vi "New.vi"(8 "Error In":errorcluster) -> (0 "Error Out":errorcluster, 3 "String":refnum<class "String.lvclass">)   [LabVIEW 2018]
uses:
  String.lvclass
  D:/Users/cfield/Code/Field R&D Services/Mustache/trunk/src/Toolkit/Writers/Abstract/Abstract.lvclass
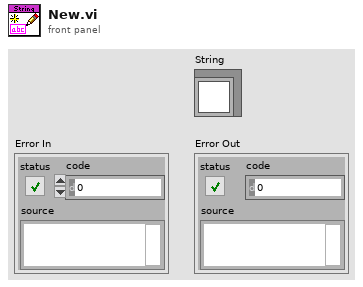
[diagram p1: front panel]
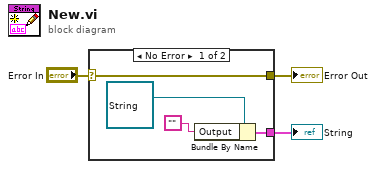
[diagram p0: block diagram]
diagram:
  n1 = case shown="No Error" "Error In" {
    selector: "Error In" -> [w4 w8]
    tunnel: [w6 _] -> w3
    tunnel: [w4 w8] -> w1
    frame No Error {
      n2 = Bundle By Name(cluster=refnum<class "String.lvclass"> refnum ("Toolkit.lvlib:Writers.lvlib:String.lvclass"), "Output"="") -> (w6:cluster{})
    }
    frame Error {
    }
  }
  "String" <- w3
  "Error Out" <- w1
